vi "Teleop.vi"(10 "Match Info":T1={"Autonomous Elapsed Seconds"=0.0, "TeleOp Elapsed Seconds"=0.0, "Disabled Elapsed Seconds"=0.0, "Visited Autonomous"=FALSE, "Visited TeleOp"=FALSE, "Visited Disabled"=FALSE, "Autonomous Settings"={"Autonomous Style"=enum."Independent", "VI Refnum"=refnum}}, 11 "Call Context":T2) -> ()   [LabVIEW 2019]
doc: "This VI is called for each TeleOp packet received from the DS where the robot is not disabled. It is often used to read from the joysticks and update I/O or to update setpoints for timed control loops. It should complete and return within 20 milliseconds or it may miss DS packets."
uses:
  <vilib>/Rock Robotics/WPI/DriverStation/WPI_DriverStationDerivedRobotMode.ctl
  <vilib>/Rock Robotics/WPI/DriverStation/WPI_DriverStationMatch Info.ctl
  <vilib>/Rock Robotics/WPI/Utilities/WPI_GetSetVariantRefNum.vi
  <vilib>/Rock Robotics/Network Tables/NT Write Boolean Array.vi
  <vilib>/Rock Robotics/Network Tables/NT Write Numeric Array.vi
  Shoot/Shoot Global.vi
  Index/Index Global.vi
  Drive/Drive Global.vi
  Climb/Climb Global.vi
  Intake/Intake Global.vi
  Vanna/Vanna Global.vi
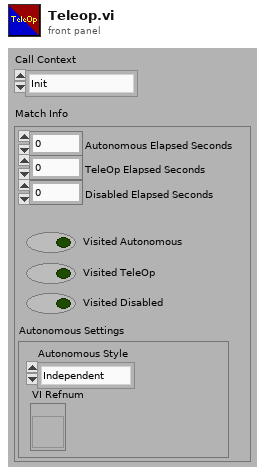
[diagram p1: front panel]
types:
  T1 = typedef "WPI_DriverStationMatch Info.ctl" = cluster{"Autonomous Elapsed Seconds":dbl, "TeleOp Elapsed Seconds":dbl, "Disabled Elapsed Seconds":dbl, "Visited Autonomous":bool, "Visited TeleOp":bool, "Visited Disabled":bool, "Autonomous Settings":cluster{"Autonomous Style":enum16{"Iterative", "Independent"}, "VI Refnum":refnum<vi>}}
  T2 = typedef "WPI_DriverStationDerivedRobotMode.ctl" = enum16{"Init", "Execute", "Stop"}
  T3 = typedef "WPI_JoystickDevRef.ctl" = cluster{"Device":T4}
  T4 = typedef "WPI_JoystickDeviceEnum.ctl" = enum16{"USB 0", "USB 1", "USB 2", "USB 3", "USB 4", "USB 5"}
  T5 = typedef "Joystick Controls.ctl" = cluster{"Driver Left Joystick X":dbl, "Driver Left Joystick Y":dbl, "Driver A Button":bool, "Driver B Button":bool, "Driver X Button":bool, "Driver Y Button":bool, "Driver Left Bumper":bool, "Driver Right Bumper":bool, "Driver View Button":bool, "Driver Menu Button":bool, "Driver Left Joystick Press":bool, "Driver Right Joystick Press":bool, "Driver Left Trigger":dbl, "Driver Right Joystick X":dbl, "Driver Right Joystick Y":dbl, "Driver Right Trigger":dbl, "Operator Left Joystick X":dbl, "Operator Left Joystick Y":dbl, "Operator A Button":bool, "Operator B Button":bool, "Operator X Button":bool, "Operator Y Button":bool, "Operator Left Bumper":bool, "Operator Right Bumper":bool, "Operator View Button":bool, "Operator Menu Button":bool, "Operator Left Joystick Press":bool, "Operator Right Joystick Press":bool, "Operator Left Trigger":dbl, "Operator Right Joystick X":dbl, "Operator Right Joystick Y":dbl, "Operator Right Trigger":dbl, "Driver D-Pad":i16, "Operator D-Pad":i16}
  T6 = typedef "Vanna Command Type Def.ctl" = cluster{"Vanna Mode":T7, "Throttle (%)":dbl, "Timestamp (ms)":dbl}
  T7 = typedef "Vanna Mode Type Def.ctl" = enum16{"Disabled", "Raw Throttle", "Rotation Control", "Position Control"}
  T8 = typedef "Intake Command Type Def.ctl" = cluster{"Intake Mode":T9, "Throttle (%)":dbl, "Pneumatic State":T10}
  T9 = typedef "Intake Mode Type Def.ctl" = enum16{"Disabled", "Enabled"}
  T10 = typedef "WPI_SolenoidValue.ctl" = enum16{"Off", "On", "Forward", "Reverse"}
  T11 = typedef "Climb Command Type Def.ctl" = cluster{"Climb Mode":T12, "Throttle (%)":dbl, "Timestamp (ms)":dbl, "Skywalker Throttle (%)":dbl}
  T12 = typedef "Climb Mode Type Def.ctl" = enum16{"Disabled", "Raw Throttle", "Auto Climb"}
  T13 = typedef "Drive Command Typedef.ctl" = cluster{"Drive Mode":T14, "LeftValue(%)/ relative Distance[u]":dbl, "Right Motor Value(%)/ absolute angle (deg)":dbl, "Timestamp (ms)":dbl}
  T14 = typedef "Drive Mode Typedef.ctl" = enum16{"Disabled", "Auto-align", "Drive Distance", "Turn to angle", "Driver"}
  T15 = typedef "Shooter Command Type Def.ctl" = cluster{"Shooter Mode":T16, "Throttle (%)/ \nSetpoint (RPM)":dbl, "Timestamp (ms)":dbl}
  T16 = typedef "Shooter Mode Type Def.ctl" = enum16{"Disabled", "Raw Throttle", "Velocity Control"}
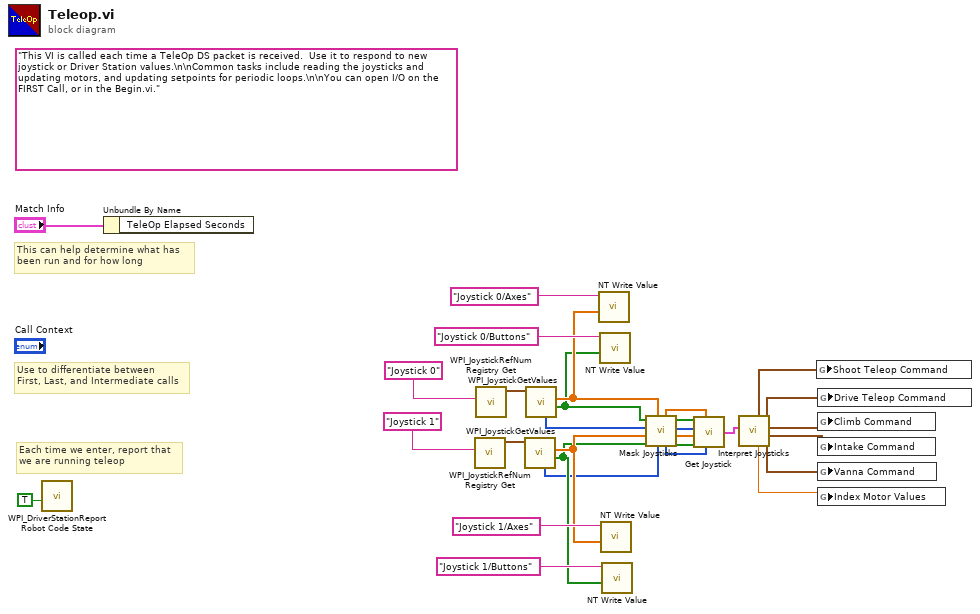
[diagram p0: block diagram]
diagram:
  (unwired) "This VI is called each time a TeleOp DS packet is received.  Use it to respond to new joystick or Driver Station values.\n\nCommon tasks include reading the joysticks and updating motors, and updating setpoints for periodic loops.\n\nYou can open I/O on the FIRST Call, or in the Begin.vi."
  # "Each time we enter, report that\nwe are running teleop"
  # "Use to differentiate between\nFirst, Last, and Intermediate calls"
  # "This can help determine what has\nbeen run and for how long"
  n1 = call <vilib>:"WPI_DriverStationReport Robot Code State.vi"("TeleOp"=TRUE ("Autonomous")) -> ()  [unwired: 10 in, 1 out]
  n2 = Unbundle By Name("Match Info") -> ()  [unwired: 1 out]
  n3 = call <vilib>:"WPI_JoystickRefNum Registry Get.vi"("refnum name"="Joystick 1") -> ("JoystickDevRef"=w22:T3)  [unwired: 1 in, 9 out]
  n4 = call <vilib>:"WPI_JoystickRefNum Registry Get.vi"("refnum name"="Joystick 0") -> ("JoystickDevRef"=w27:T3)  [unwired: 1 in, 9 out]
  n5 = call <vilib>:"WPI_JoystickGetValues.vi"("JoystickDevRef"=w22) -> ("Buttons"=w15:bool[], "Axes"=w16:dbl[], "POVs"=w14:i16[])  [unwired: 6 in, 2 out]
  n6 = call <vilib>:"WPI_JoystickGetValues.vi"("JoystickDevRef"=w27) -> ("Buttons"=w18:bool[], "Axes"=w19:dbl[], "POVs"=w17:i16[])  [unwired: 6 in, 2 out]
  n7 = call-poly <vilib>:"NT Write Value.vi"("Numeric Array"=w19, "Name"="Joystick 0/Axes") -> ()  [unwired: 9 in, 1 out]
  n8 = call-poly <vilib>:"NT Write Value.vi"("Boolean Array"=w18, "Name"="Joystick 0/Buttons") -> ()  [unwired: 9 in, 1 out]
  n9 = call-poly <vilib>:"NT Write Value.vi"("Numeric Array"=w16, "Name"="Joystick 1/Axes") -> ()  [unwired: 9 in, 1 out]
  n10 = call-poly <vilib>:"NT Write Value.vi"("Boolean Array"=w15, "Name"="Joystick 1/Buttons") -> ()  [unwired: 9 in, 1 out]
  n11 = call "Mask Joysticks.vi"("Operator POVs"=w14, "Driver Axes"=w19, "Operator Buttons"=w15, "Operator Axes"=w16, "Driver POVs"=w17, "Driver Buttons"=w18) -> ("Operator Buttons Out"=w9:bool[], "Operator Axes Out"=w10:dbl[], "Driver POVs Out"=w11:i16[], "Drive Buttons Out"=w12:bool[], "Operator POVs Out"=w8:i16[], "Drive Axes Out"=w13:dbl[])
  n12 = call "Get Joystick.vi"("Operator POVs"=w8, "Driver Axes"=w13, "Operator Buttons"=w9, "Operator Axes"=w10, "Driver POVs"=w11, "Driver Buttons"=w12) -> ("Joystick Controls Out"=w7:T5)
  n13 = call "Interpret Joysticks.vi"("Joystick Controls"=w7) -> ("Vanna Teleop Command"=w3:T6, "Intake Teleop Command"=w4:T8, "Climb Teleop Command"=w5:T11, "Drive Teleop command"=w6:T13, "Index Teleop Command"=w2:dbl, "Shoot Teleop Command"=w1:T15)  [unwired: 5 in]
  n14 = global write "Shoot Global.vi" "Shoot Teleop Command"(w1) -> ()
  n15 = global write "Drive Global.vi" "Drive Teleop Command"(w6) -> ()
  n16 = global write "Climb Global.vi" "Climb Command"(w5) -> ()
  n17 = global write "Intake Global.vi" "Intake Command"(w4) -> ()
  n18 = global write "Vanna Global.vi" "Vanna Command"(w3) -> ()
  n19 = global write "Index Global.vi" "Index Motor Values"(w2) -> ()
